vi "n58_manual_status.vi"(8 "error in (no error)":errorcluster, 10 "Research exe":string="\"D:\\River\\DTU_EOL_24\\EXEs\\RESEARCHDOWNLOAD_R22.19.1701\\RESEARCHDOWNLOAD_R22.19.1701_DUT1\\Bin\\ResearchDownload.exe\"", 11 "DUT":string) -> (0 "error out":errorcluster, 2 "Status":string)   [LabVIEW 2024]
panel:
  out "DUT":string
  in  "FAIL":bool
  in  "success":bool
  # "N58 FLASH"
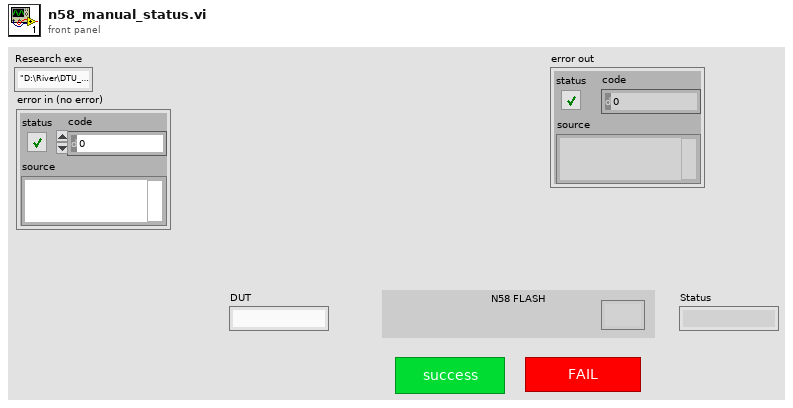
[diagram p1: front panel]
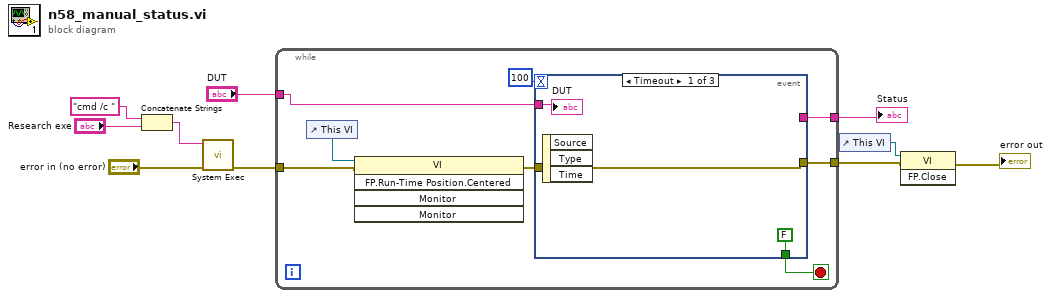
[diagram p0: block diagram]
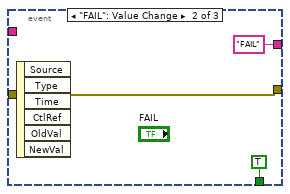
[diagram p2: hidden frame]
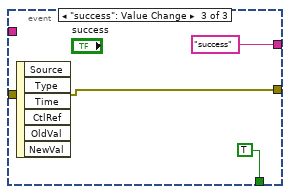
[diagram p3: hidden frame]
diagram:
  n1 = Concatenate Strings("cmd /c ", "Research exe") -> (w8:string)
  n2 = call <vilib>:"System Exec.vi"("error in (no error)"="error in (no error)", "command line"=w8) -> ("error out"=w6:errorcluster)  [unwired: 6 in, 3 out]
  n3 = while {
    tunnel: w6 -> [w13]
    tunnel: [w17] -> w3
    tunnel: [w16] -> w5
    tunnel: "DUT" -> [w11]
    stop <- w15 stop-if-true
    n4 = control-ref of="This VI"() -> (w14:refnum<vi>)
    n5 = invoke class="VI" method="FP.Run-Time Position.Centered"(reference=w14, error in=w13) -> (error out=w12:errorcluster)  [unwired: 3 in, 4 out]
    n6 = event shown="[0] Timeout" {
      selector: _ -> [_ _ _]
      dyn-events: _ -> [_ _ _]
      timeout: 100 -> [_ _ _]
      tunnel: w12 -> [w21 w24 w27]
      tunnel: [w21 w24 w27] -> w17
      tunnel: [_ "FAIL" "success"] -> w16
      tunnel: [FALSE TRUE TRUE] -> w15
      tunnel: w11 -> [w19 _ _]
      event Timeout {
        n7 = event-data() -> ()  [unwired: 1 in, 3 out]
        "DUT" <- w19
      }
      event "FAIL": Value Change {
        n8 = event-data() -> ()  [unwired: 1 in, 6 out]
      }
      event "success": Value Change {
        n9 = event-data() -> ()  [unwired: 1 in, 6 out]
      }
    }
  }
  "Status" <- w5
  n10 = control-ref of="This VI"() -> (w4:refnum<vi>)
  n11 = invoke class="VI" method="FP.Close"(reference=w4, error in=w3) -> (error out=→"error out":errorcluster)  [unwired: 1 in, 2 out]
